vi "JSONRPC-ArrayToString_Poly.vi"   [LabVIEW 2020]
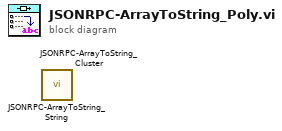
[diagram p0: block diagram]
diagram:
  n1 = call "JSONRPC-ArrayToString_String.vi"() -> ()  [unwired: 11 in, 1 out]
  n2 = call "JSONRPC-ArrayToString_Cluster.vi"() -> ()  [unwired: 11 in, 1 out]
